vi "BoP.vi"() -> ()   [LabVIEW 2017]
panel:
  in  "Stop":bool
  in  "NG Flow Rate":sgl=418.0
  in  "CTAH 2 Heat Input":sgl=418.0
  in  "CTAH 1 Heat Input":sgl=418.0
  out "Compressor Work":sgl=1000000.0
  in  "Shaft RPM [x1000]":sgl=418.0
  out "Mass Flow":sgl(graph)
  out "Turbine Work Output":sgl[](graph)
  out "P1":sgl format="%.1f"
  out "T1":sgl format="%.1f"
  out "P2":sgl format="%.1f"
  out "T2":sgl format="%.1f"
  out "P3":sgl format="%.1f"
  out "T3":sgl format="%.1f"
  out "P4":sgl format="%.1f"
  out "T4":sgl format="%.1f"
  out "P5":sgl format="%.1f"
  out "T5":sgl format="%.1f"
  out "P6":sgl format="%.1f"
  out "T6":sgl format="%.1f"
  out "HPT Work Output":sgl=1000000.0
  out "LPT Work Output":sgl=137940000.0
  out "Pressure Drop 1st Pass":sgl format="%#.1g"
  out "Pressure Drop 2nd pass":sgl format="%#.1g"
  # "Balance of Plant"
  # "Trends and Analytics"
  # "HIGH PRESSURE\nTURBINE"
  # "LOW PRESSURE\nTURBINE"
  # "COMPRESSOR"
  # "CTAH"
  # "Temperatures in K\nPressures in Pa"
  # "Load and Demand"
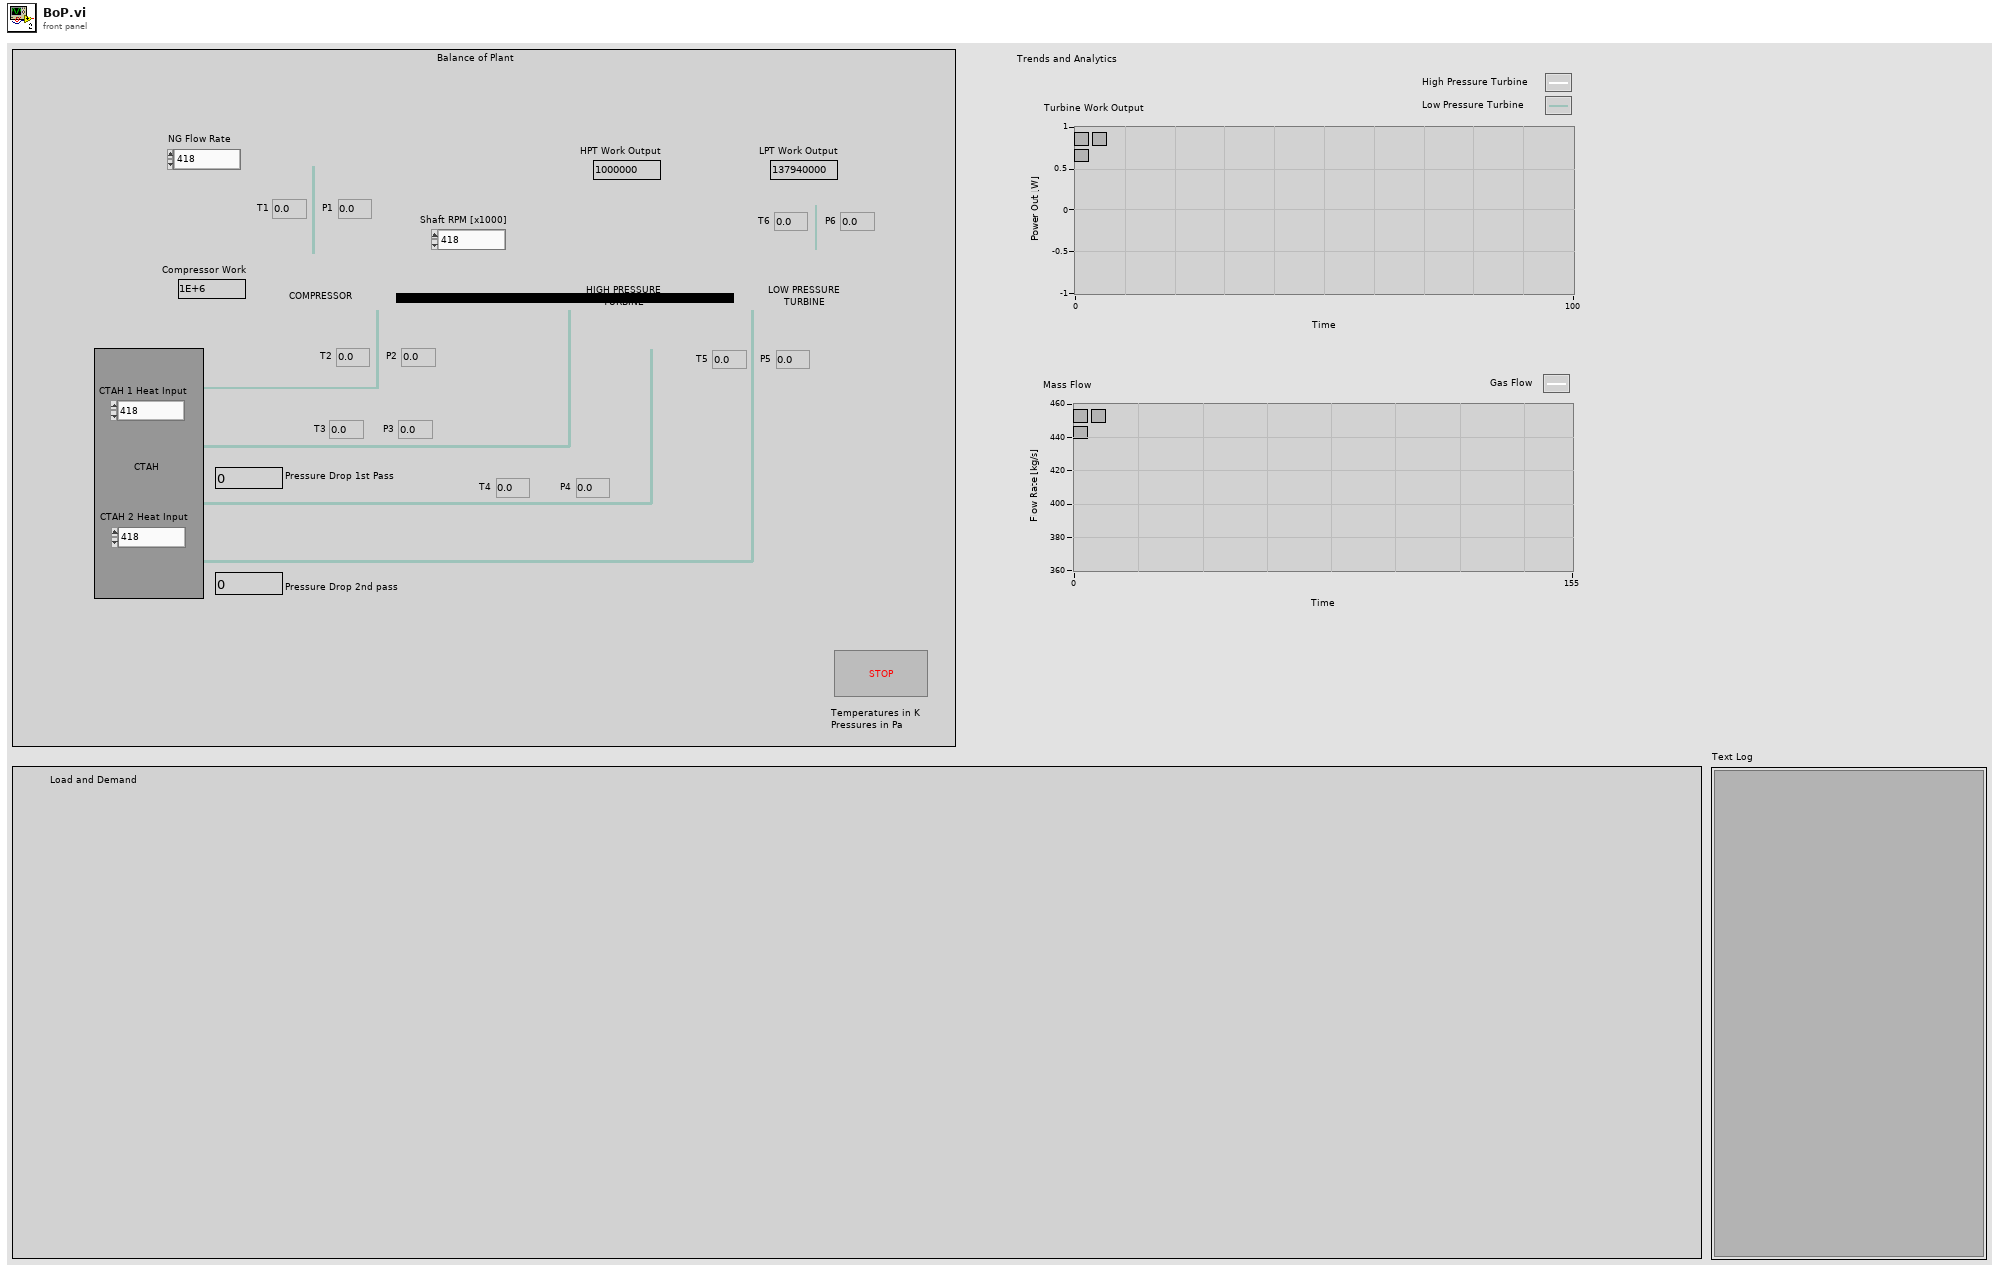
[diagram p1: front panel]
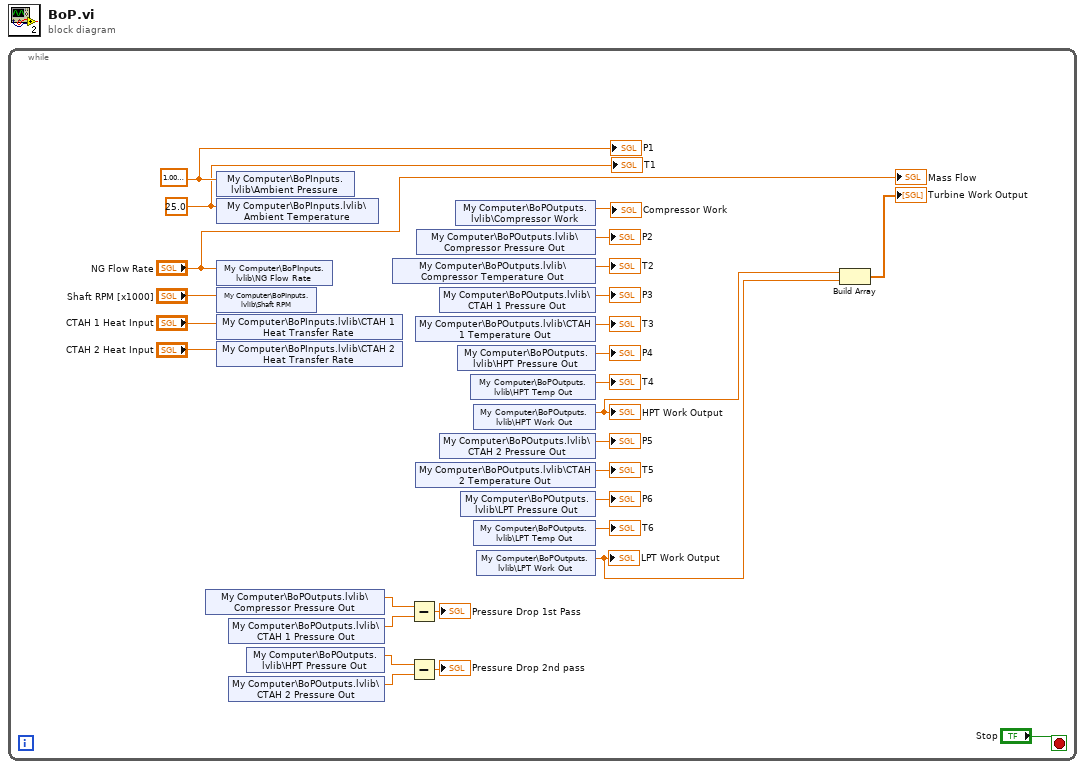
[diagram p0: block diagram]
diagram:
  n1 = while {
    stop <- "Stop" stop-if-true
    w23 = sgl 25.0 ("Incoming Air Temp")
    w24 = sgl 1.01 ("Incoming Air Pressure")
    n2 = shared-variable "My Computer\\BoPOutputs.lvlib\\Compressor Pressure Out"() -> (w6:sgl)  [unwired: 1 in, 1 out]
    n3 = shared-variable "My Computer\\BoPInputs.lvlib\\Ambient Pressure"(w24) -> ()  [unwired: 1 in, 1 out]
    n4 = shared-variable "My Computer\\BoPInputs.lvlib\\Ambient Temperature"(w23) -> ()  [unwired: 1 in, 1 out]
    n5 = shared-variable "My Computer\\BoPInputs.lvlib\\NG Flow Rate"("NG Flow Rate") -> ()  [unwired: 1 in, 1 out]
    n6 = shared-variable "My Computer\\BoPInputs.lvlib\\Shaft RPM"("Shaft RPM [x1000]") -> ()  [unwired: 1 in, 1 out]
    n7 = shared-variable "My Computer\\BoPInputs.lvlib\\CTAH 1 Heat Transfer Rate"("CTAH 1 Heat Input") -> ()  [unwired: 1 in, 1 out]
    n8 = shared-variable "My Computer\\BoPInputs.lvlib\\CTAH 2 Heat Transfer Rate"("CTAH 2 Heat Input") -> ()  [unwired: 1 in, 1 out]
    n9 = shared-variable "My Computer\\BoPOutputs.lvlib\\CTAH 1 Pressure Out"() -> (w5:sgl)  [unwired: 1 in, 1 out]
    n10 = shared-variable "My Computer\\BoPOutputs.lvlib\\CTAH 2 Pressure Out"() -> (w3:sgl)  [unwired: 1 in, 1 out]
    n11 = shared-variable "My Computer\\BoPOutputs.lvlib\\HPT Pressure Out"() -> (w4:sgl)  [unwired: 1 in, 1 out]
    n12 = shared-variable "My Computer\\BoPOutputs.lvlib\\Compressor Temperature Out"() -> (→"T2":sgl)  [unwired: 1 in, 1 out]
    n13 = Subtract(x=w6, y=w5) -> (x-y=→"Pressure Drop 1st Pass":sgl)
    n14 = Subtract(x=w4, y=w3) -> (x-y=→"Pressure Drop 2nd pass":sgl)
    n15 = shared-variable "My Computer\\BoPOutputs.lvlib\\CTAH 1 Temperature Out"() -> (→"T3":sgl)  [unwired: 1 in, 1 out]
    n16 = shared-variable "My Computer\\BoPOutputs.lvlib\\CTAH 2 Temperature Out"() -> (→"T5":sgl)  [unwired: 1 in, 1 out]
    n17 = shared-variable "My Computer\\BoPOutputs.lvlib\\Compressor Pressure Out"() -> (→"P2":sgl)  [unwired: 1 in, 1 out]
    n18 = shared-variable "My Computer\\BoPOutputs.lvlib\\CTAH 1 Pressure Out"() -> (→"P3":sgl)  [unwired: 1 in, 1 out]
    n19 = shared-variable "My Computer\\BoPOutputs.lvlib\\CTAH 2 Pressure Out"() -> (→"P5":sgl)  [unwired: 1 in, 1 out]
    n20 = shared-variable "My Computer\\BoPOutputs.lvlib\\Compressor Work"() -> (→"Compressor Work":sgl)  [unwired: 1 in, 1 out]
    n21 = shared-variable "My Computer\\BoPOutputs.lvlib\\HPT Pressure Out"() -> (→"P4":sgl)  [unwired: 1 in, 1 out]
    n22 = shared-variable "My Computer\\BoPOutputs.lvlib\\LPT Pressure Out"() -> (→"P6":sgl)  [unwired: 1 in, 1 out]
    n23 = shared-variable "My Computer\\BoPOutputs.lvlib\\HPT Temp Out"() -> (→"T4":sgl)  [unwired: 1 in, 1 out]
    n24 = shared-variable "My Computer\\BoPOutputs.lvlib\\HPT Work Out"() -> (w2:sgl)  [unwired: 1 in, 1 out]
    "HPT Work Output" <- w2
    n25 = shared-variable "My Computer\\BoPOutputs.lvlib\\LPT Temp Out"() -> (→"T6":sgl)  [unwired: 1 in, 1 out]
    n26 = shared-variable "My Computer\\BoPOutputs.lvlib\\LPT Work Out"() -> (w12:sgl)  [unwired: 1 in, 1 out]
    "LPT Work Output" <- w12
    n27 = Build Array(w2, w12) -> (→"Turbine Work Output":sgl[])
    "P1" <- w24
    "T1" <- w23
    "Mass Flow" <- "NG Flow Rate"
  }
